vi "Set Freq Sweep Stop.vi"(8 "error in (no error)":errorcluster, 10 "Frequency Sweep Stop":dbl[unit], 11 "VISA resource name":refnum<visa-resource-name>) -> (0 "error out":errorcluster, 3 "VISA resource name out":refnum<visa-resource-name>)   [LabVIEW 2009, in "Agilent PSG MXG Series.lvlib"]
uses:
  Agilent PSG MXG Series.lvlib
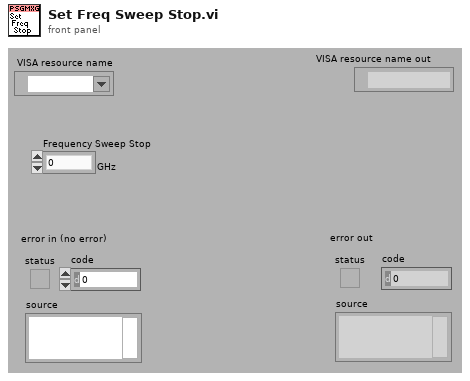
[diagram p1: front panel]
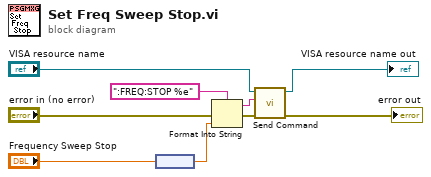
[diagram p0: block diagram]
diagram:
  n1 = node("Frequency Sweep Stop") -> (w2:dbl)
  n2 = Format Into String(format string=":FREQ:STOP %e", error in="error in (no error)", w2) -> (resulting string=w3:string, error out=w4:errorcluster)  [unwired: 1 in]
  n3 = call "Send Command.vi"("error in (no error)"=w4, "write buffer"=w3, "VISA resource name"="VISA resource name") -> ("error out"=→"error out":errorcluster, "VISA resource name out"=→"VISA resource name out":refnum<visa-resource-name>)  [unwired: 7 out]
